vi "FRCts20_Backend_Test_RequestRoot_GET.vi"(8 "error in (no error)":errorcluster) -> (0 "error out":errorcluster, 1 "Time (ms)":u32, 2 "Status":string, 5 "Success":bool)   [LabVIEW 2014, in "FRCts20_Backend_TestCode.lvlib"]
uses:
  FRCts20_Backend_TestCode.lvlib
  FRCts20_Backend_API/FRCts20_Backend_API_RequestRoot.vi
  FRCts20_Backend_API/FRCts20_Backend_API_Status.ctl
  FRCts20_Backend_API/FRCts20_Backend_API_RequestRoot.ctl
  FRCts20_Backend_API/FRCts20_Backend_API_Command_RequestRoot.ctl
panel:
  out "Request Out":T1
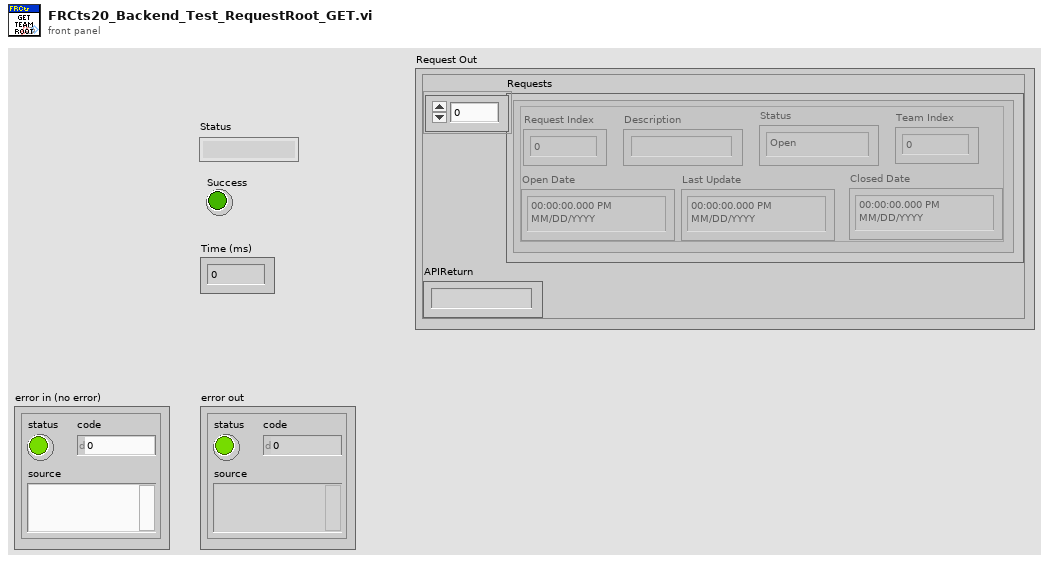
[diagram p1: front panel]
types:
  T1 = typedef "FRCts20_Backend_API.lvlib/FRCts20_Backend_API_RequestRoot.ctl" = cluster{"Requests":cluster{"Request Index":u32, "Description":string, "Status":T2, "Open Date":timestamp, "Last Update":timestamp, "Closed Date":timestamp, "Team Index":u32}[], "APIReturn":string}
  T2 = typedef "FRCts20_Backend_API.lvlib/FRCts20_Backend_API_Status.ctl" = enum16{"Open", "In Work", "Closed"}
  T3 = typedef "FRCts20_Backend_API.lvlib/FRCts20_Backend_API_Command_RequestRoot.ctl" = string
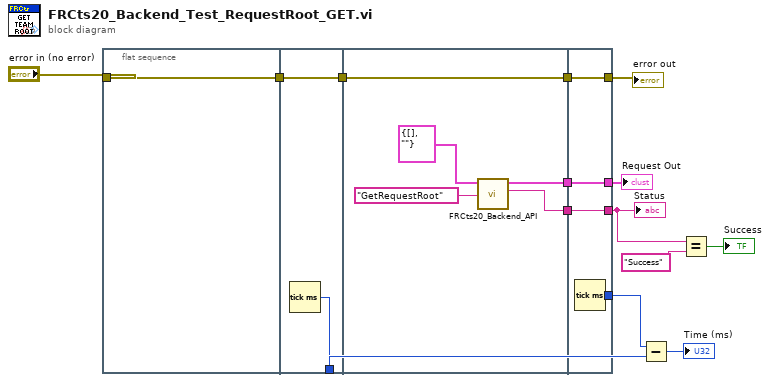
[diagram p0: block diagram]
diagram:
  n1 = flat-sequence {
    tunnel: "error in (no error)" -> [w15]
    tunnel: [w15] -> w14
    tunnel: [w17] -> w4
    tunnel: [w16] -> w13
    tunnel: w14 -> [w16]
    tunnel: [w22] -> w12
    tunnel: w13 -> [w22]
    tunnel: [w21] -> w11
    tunnel: [w20] -> w2
    tunnel: [w26] -> w5
    tunnel: [w25] -> w7
    tunnel: w12 -> [w25]
    tunnel: [w24] -> w3
    tunnel: w11 -> [w24]
    tunnel: [w23] -> w1
    tunnel: w2 -> [w23]
    frame #0 {
    }
    frame #1 {
      n2 = Tick Count (ms)() -> (millisecond timer value=w17:u32)
    }
    frame #2 {
      n3 = call-poly "FRCts20_Backend_API.vi"("Message"=T3 "GetRequestRoot", "Request In"=T1 {"Requests"=[], "APIReturn"=""}) -> ("Status"=w21:string, "Request Out"=w20:T1)  [unwired: 7 in, 1 out]
    }
    frame #3 {
      n4 = Tick Count (ms)() -> (millisecond timer value=w26:u32)
    }
  }
  n5 = Subtract(x=w5, y=w4) -> (x-y=→"Time (ms)":u32)
  n6 = Equal?(x=w3, y="Success") -> (x = y?=→"Success":bool)
  "Status" <- w3
  "error out" <- w7
  "Request Out" <- w1
